vi "DC Pulses Blocks with Ramps.vi"() -> ()   [LabVIEW 2020]
uses:
  <vilib>/Analysis/1siggen.llb/Ramp Pattern by Samples.vi
  <vilib>/DAQmx/write.llb/DAQmx Write (Analog Wfm 1Chan NSamp).vi
  <vilib>/Waveform/WDTOps.llb/WDT Append Waveforms DBL.vi
  <vilib>/Waveform/WDTOps.llb/WDT Number of Waveform Samples DBL.vi
  <vilib>/DAQmx/create/channels.llb/DAQmx Create Channel (AO-Voltage-Basic).vi
  <vilib>/DAQmx/configure/timing.llb/DAQmx Timing (Use Waveform).vi
  <vilib>/DAQmx/miscellaneous.llb/DAQmx Fill In Error Info.vi
  <vilib>/measure/NI_MAPro.lvlib
  <vilib>/Analysis/NI_AALBase.lvlib
  <resource>/objmgr/daqmx.rc
panel:
  out "Loop?":bool=TRUE
  in  "Stop":bool
  in  "DAQ Output Channel":tag
  in  "Full Ramp\nTime (sec)":dbl=0.02 min=1.0
  out "Output Waveform":waveform(dbl)(graph)
  out "Total Time (s)":dbl
  in  "Second Pulse\nTime (sec)":dbl=1.0 min=1.0
  in  "Second Pulse\nAmplitude (mA)":dbl min=-10.0 max=10.0
  in  "First Pulse\nTime (sec)":dbl=1.0 min=1.0
  in  "First Pulse\nAmplitude (mA)":dbl min=-10.0 max=10.0
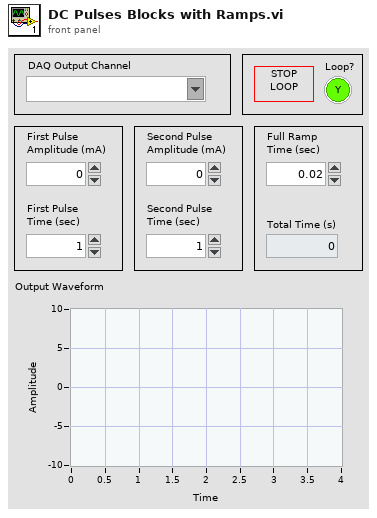
[diagram p1: front panel]
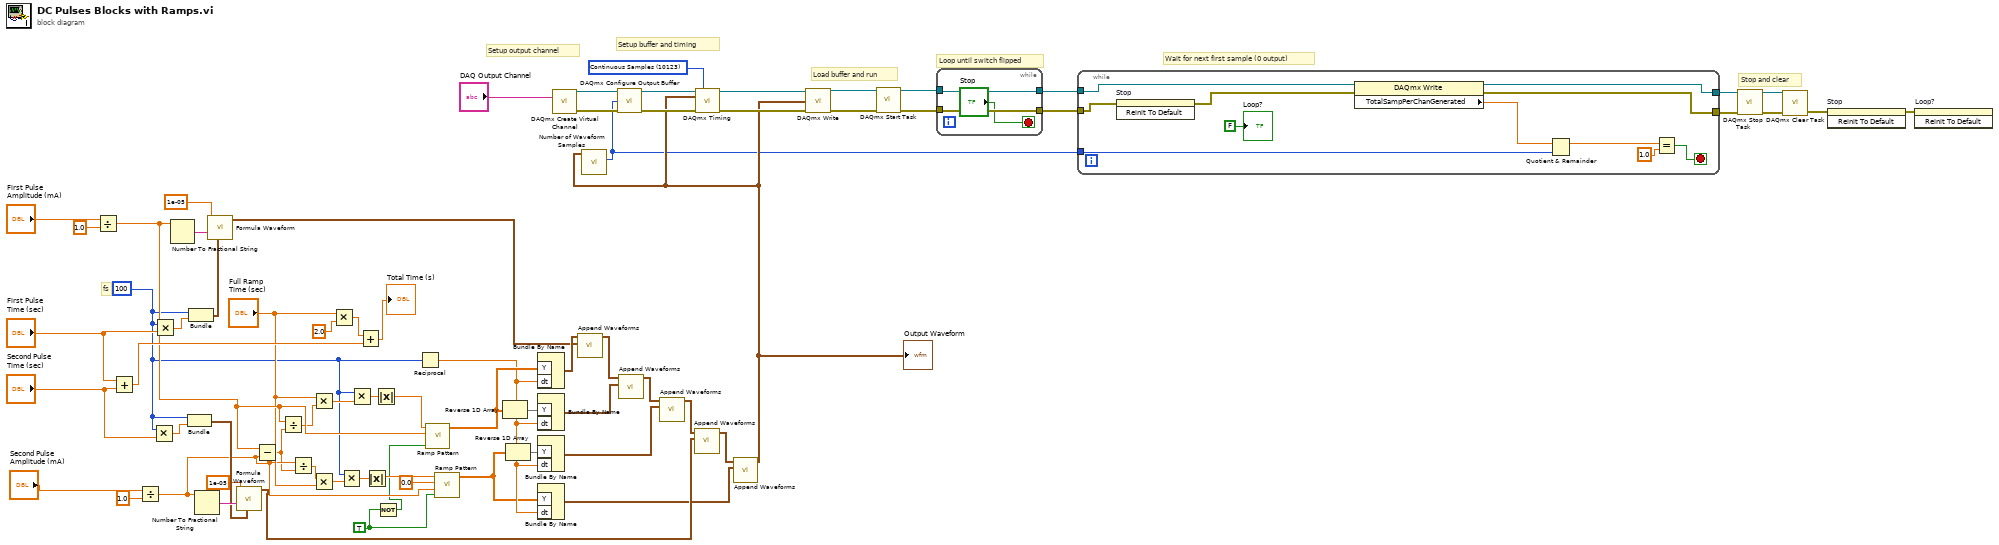
[diagram p0: block diagram]
diagram:
  w8 = 10123 items=["Finite Samples"=10178, "Continuous Samples"=10123, "Hardware Timed Single Point"=12522] ("sample mode")
  w24 = TRUE ("exclude end?")
  w48 = u32 100
  # "Load buffer and run"
  # "Setup buffer and timing"
  # "Setup output channel"
  # "Stop and clear"
  # "Wait for next first sample (0 output)"
  # "Loop until switch flipped"
  # "fs"
  n1 = Divide(x="First Pulse\nAmplitude (mA)", y=1.0) -> (x/y=w53:dbl)
  n2 = Add(x="First Pulse\nTime (sec)", y="Second Pulse\nTime (sec)") -> (x+y=w56:dbl)
  n3 = Divide(x="Second Pulse\nAmplitude (mA)", y=1.0) -> (x/y=w46:dbl)
  n4 = Multiply(x=w48, y="Second Pulse\nTime (sec)") -> (x*y=w70:dbl)
  n5 = Multiply(x=w48, y="First Pulse\nTime (sec)") -> (x*y=w71:dbl)
  n6 = Number To Fractional String(number=w53) -> (F-format string=w69:string)  [unwired: 3 in]
  n7 = Bundle(w48, w70) -> (w66:cluster{u32, dbl})  [unwired: 1 in]
  n8 = Bundle(w48, w71) -> (w68:cluster{u32, dbl})  [unwired: 1 in]
  n9 = Number To Fractional String(number=w46) -> (F-format string=w67:string)  [unwired: 3 in]
  n10 = call <vilib>:"Formula Waveform.vi"("sampling info"=w68, "formula"=w69, "frequency"=1e-05) -> ("signal out"=w44:waveform(dbl))  [unwired: 7 in, 1 out]
  n11 = call <vilib>:"Formula Waveform.vi"("sampling info"=w66, "formula"=w67, "frequency"=1e-05) -> ("signal out"=w35:waveform(dbl))  [unwired: 7 in, 1 out]
  n12 = Subtract(x=w53, y=w46) -> (x-y=w30:dbl)
  n13 = Divide(x=w53, y=w30) -> (x/y=w52:dbl)
  n14 = Divide(x=w46, y=w30) -> (x/y=w49:dbl)
  n15 = Multiply(x="Full Ramp\nTime (sec)", y=w52) -> (x*y=w51:dbl)
  n16 = Multiply(x=w49, y="Full Ramp\nTime (sec)") -> (x*y=w47:dbl)
  n17 = Multiply(x="Full Ramp\nTime (sec)", y=2.0) -> (x*y=w55:dbl)
  n18 = Multiply(x=w48, y=w47) -> (x*y=w27:dbl)
  n19 = Multiply(x=w48, y=w51) -> (x*y=w29:dbl)
  n20 = Add(x=w55, y=w56) -> (x+y=→"Total Time (s)":dbl)
  n21 = Absolute Value(x=w27) -> (abs(x)=w26:dbl)
  n22 = Absolute Value(x=w29) -> (abs(x)=w28:dbl)
  n23 = Not(x=w24) -> (.not. x?=w23:bool)
  n24 = Reciprocal(x=w48) -> (1/x=w40:dbl)
  n25 = call-poly <vilib>:"Ramp Pattern.vi"("exclude end?"=w23, "end"=w53, "samples"=w28) -> ("Ramp Pattern"=w41:dbl[])  [unwired: 7 in, 1 out]
  n26 = call-poly <vilib>:"Ramp Pattern.vi"("exclude end?"=w24, "start"=w46, "end"=0.0, "samples"=w26) -> ("Ramp Pattern"=w32:dbl[])  [unwired: 6 in, 1 out]
  n27 = Reverse 1D Array(array=w41) -> (reversed array=w42:dbl[])
  n28 = Reverse 1D Array(array=w32) -> (reversed array=w31:dbl[])
  n29 = Bundle By Name("Y"=w41, "dt"=w40) -> (w45:waveform(dbl))  [unwired: 1 in]
  n30 = Bundle By Name("Y"=w42, "dt"=w40) -> (w39:waveform(dbl))  [unwired: 1 in]
  n31 = Bundle By Name("Y"=w31, "dt"=w40) -> (w37:waveform(dbl))  [unwired: 1 in]
  n32 = Bundle By Name("Y"=w32, "dt"=w40) -> (w33:waveform(dbl))  [unwired: 1 in]
  n33 = call-poly <vilib>:"DAQmx Create Virtual Channel.vi"("physical channels"="DAQ Output Channel") -> ("task out"=w11:refnum<k21>, "error out"=w10:errorcluster)  [unwired: 13 in]
  n34 = call-poly <vilib>:"Append Waveforms.vi"("waveform B"=w44, "waveform A"=w45) -> ("waveform out"=w43:waveform(dbl))  [unwired: 8 in, 1 out]
  n35 = call-poly <vilib>:"Append Waveforms.vi"("waveform B"=w39, "waveform A"=w43) -> ("waveform out"=w38:waveform(dbl))  [unwired: 8 in, 1 out]
  n36 = call-poly <vilib>:"Append Waveforms.vi"("waveform B"=w37, "waveform A"=w38) -> ("waveform out"=w36:waveform(dbl))  [unwired: 8 in, 1 out]
  n37 = call-poly <vilib>:"Append Waveforms.vi"("waveform B"=w35, "waveform A"=w36) -> ("waveform out"=w34:waveform(dbl))  [unwired: 8 in, 1 out]
  n38 = call-poly <vilib>:"Append Waveforms.vi"("waveform B"=w33, "waveform A"=w34) -> ("waveform out"=w9:waveform(dbl))  [unwired: 8 in, 1 out]
  "Output Waveform" <- w9
  n39 = call-poly <vilib>:"Number of Waveform Samples.vi"("waveform in"=w9) -> ("number of samples"=w3:i32)  [unwired: 8 in, 2 out]
  n40 = call <vilib>:"DAQmx Configure Output Buffer.vi"("task/channels in"=w11, "buffer size (in samples per channel)"=w3, "error in"=w10) -> ("task out"=w13:refnum<k21>, "error out"=w12:errorcluster)  [unwired: 11 in]
  n41 = call-poly <vilib>:"DAQmx Timing.vi"("task/channels in"=w13, "sample mode"=w8, "waveform"=w9, "error in"=w12) -> ("task out"=w19:refnum<k21>, "error out"=w18:errorcluster)  [unwired: 10 in]
  n42 = call-poly <vilib>:"DAQmx Write.vi"("task/channels in"=w19, "data"=w9, "error in"=w18) -> ("task out"=w21:refnum<k21>, "error out"=w20:errorcluster)  [unwired: 10 in, 1 out]
  n43 = call <vilib>:"DAQmx Start Task.vi"("task/channels in"=w21, "error in"=w20) -> ("task out"=w17:refnum<k21>, "error out"=w16:errorcluster)  [unwired: 12 in]
  n44 = while {
    tunnel: w17 -> [w74]
    tunnel: w16 -> [w73]
    tunnel: [w74] -> w4
    tunnel: [w73] -> w7
    stop <- "Stop" stop-if-true
  }
  n45 = while {
    tunnel: w4 -> [w85]
    tunnel: w7 -> [w77]
    tunnel: [w83] -> w6
    tunnel: [w84] -> w5
    tunnel: w3 -> [w82]
    stop <- w78 stop-if-true
    n46 = invoke on="Stop" class="Bool" method="Reinit To Default"(error in=w77) -> (error out=w76:errorcluster)  [unwired: 2 in, 2 out]
    n47 = property class="DAQmx Write"(reference=w85, error in=w76) -> (reference out=w83:refnum<k21>, error out=w84:errorcluster, "TotalSampPerChanGenerated"=w81:dbl)
    n48 = Quotient & Remainder(x=w81, y=w82) -> (x-y*floor(x/y)=w80:dbl)  [unwired: 1 out]
    n49 = Equal?(x=w80, y=1.0) -> (x = y?=w78:bool)
    "Loop?" <- FALSE ("Loop?")
  }
  n50 = call <vilib>:"DAQmx Stop Task.vi"("task/channels in"=w6, "error in"=w5) -> ("task out"=w15:refnum<k21>, "error out"=w14:errorcluster)  [unwired: 12 in]
  n51 = call <vilib>:"DAQmx Clear Task.vi"("task in"=w15, "error in"=w14) -> ("error out"=w2:errorcluster)  [unwired: 13 in]
  n52 = invoke on="Stop" class="Bool" method="Reinit To Default"(error in=w2) -> (error out=w1:errorcluster)  [unwired: 2 in, 2 out]
  n53 = invoke on="Loop?" class="Bool (strict)" method="Reinit To Default"(error in=w1) -> ()  [unwired: 2 in, 3 out]
